vi "Matlab Param Array to I32 Array.vi"(8 "error in (no error)":errorcluster, 10 "Name":string, 11 "Matlab Param Array":cluster{"Name":string, "Data":variant}[](array[cluster])) -> (0 "error out":errorcluster, 3 "data":i32[][](array[numeric]))   [LabVIEW 2010, in "Matlab API.lvlib"]
uses:
  Matlab API.lvlib
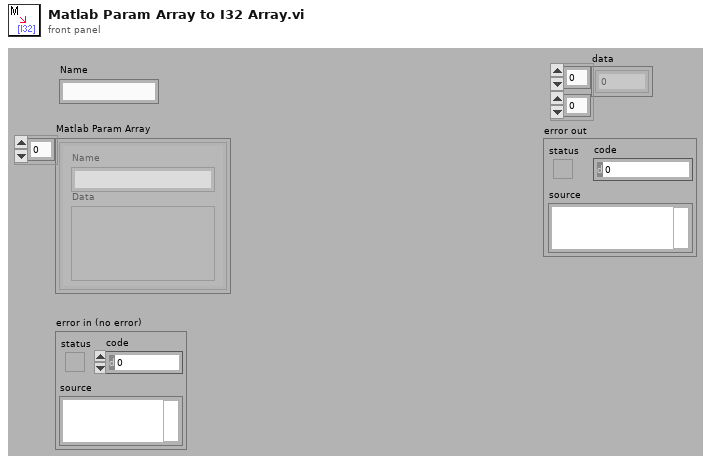
[diagram p1: front panel]
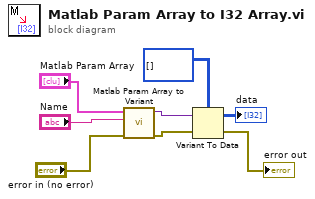
[diagram p0: block diagram]
diagram:
  n1 = call "Matlab Param Array to Variant.vi"("error in (no error)"="error in (no error)", "Name"="Name", "Variables"="Matlab Param Array") -> ("error out"=w7:errorcluster, "Data"=w8:variant)  [unwired: 7 out]
  n2 = Variant To Data(error in=w7, Variant=w8, type=i32[][] []) -> (error out=→"error out":errorcluster, data=→"data":i32[][])
